vi "Push Open.vi"(10 "node ref in":refnum<data-value>, 11 "AD* in":refnum<class "NI_Robotics_AnytimeDStar.lvclass">) -> (2 "node ref out":refnum<data-value>, 3 "AD* out":refnum<class "NI_Robotics_AnytimeDStar.lvclass">)   [LabVIEW 2017, in "NI_Robotics_AnytimeDStar.lvclass"]
uses:
  <vilib>/robotics/Navigation/Anytime D Star/NI_Robotics_AnytimeDStar.lvclass
  <vilib>/robotics/Navigation/shared/MapNode/AbstractDstarNode/NI_Robotics_AbstractDstarNode.lvclass
  c:/Program Files (x86)/National Instruments/LabVIEW 2017/vi.lib/robotics/Navigation/shared/MapNode/AbstractMapNode/NI_Robotics_AbstractMapNode.lvclass
  <vilib>/robotics/Navigation/Anytime D Star/NI_Robotics_AnytimeDStar.lvclass/NI_Robotics_AnytimeDStar.ctl
  <vilib>/robotics/Navigation/shared/Priority Queue/Open List Element.ctl
  <vilib>/robotics/Navigation/shared/MapNode/AbstractMapNode/NI_Robotics_AbstractMapNode.lvclass
  <vilib>/robotics/Navigation/shared/Priority Queue/NI_Robotics_Priority Queue.lvclass
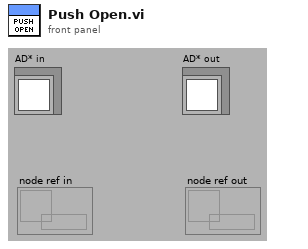
[diagram p1: front panel]
types:
  T1 = typedef "NI_Robotics_Priority Queue.lvclass/Open List Element.ctl" = cluster{"f":dbl, "g":dbl, "node Ref":refnum<data-value>}
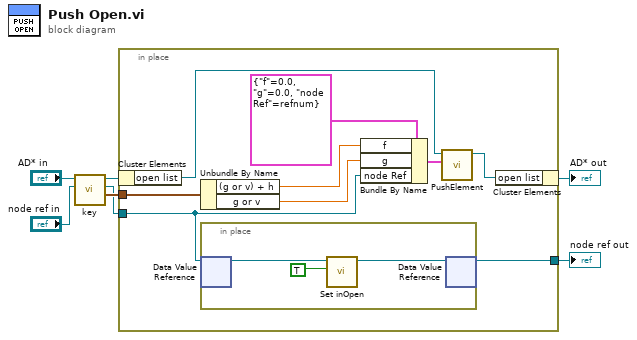
[diagram p0: block diagram]
diagram:
  n1 = call <vilib>:"key.vi"("node ref in"="node ref in", "adstar in"="AD* in") -> ("key out"=w4:cluster{"(g or v) + h":dbl, "g or v":dbl}, "node ref out"=w2:refnum<data-value>, "adstar out"=w5:refnum<class "NI_Robotics_AnytimeDStar.lvclass">)  [unwired: 7 in]
  n2 = in-place {
    in-place-border: w4 -> [w12]
    in-place-border: w2 -> [w9]
    in-place-border: [w8] -> w1
    n3 = in-place-cluster #1(w5) -> ("open list"=w14:refnum<class "NI_Robotics_Priority Queue.lvclass">)
    n4 = Unbundle By Name(w12) -> ("(g or v) + h"=w11:dbl, "g or v"=w10:dbl)
    n5 = in-place {
      n6 = in-place-dvr #2(w9) -> (w18:refnum<class "NI_Robotics_AbstractDstarNode.lvclass">)  [unwired: 1 out]
      n7 = call <vilib>:"Set inOpen.vi"("inOpen"=TRUE, "AbstractDstarNode in"=w18) -> ("AbstractDstarNode out"=w17:refnum<class "NI_Robotics_AbstractDstarNode.lvclass">)  [unwired: 8 in, 1 out]
      n8 = in-place-dvr #2(w17) -> (w8:refnum<data-value>)  [unwired: 1 out]
    }
    n9 = Bundle By Name(cluster=T1 {"f"=0.0, "g"=0.0, "node Ref"=refnum} ("Open List Element"), "f"=w11, "g"=w10, "node Ref"=w9) -> (w16:T1)
    n10 = call <vilib>:"PushElement.vi"("open list element"=w16, "Astar Open List in"=w14) -> ("Astar Open List out"=w13:refnum<class "NI_Robotics_Priority Queue.lvclass">)  [unwired: 8 in, 1 out]
    n11 = in-place-cluster #1("open list"=w13) -> (→"AD* out":refnum<class "NI_Robotics_AnytimeDStar.lvclass">)
  }
  "node ref out" <- w1
